vi "arduinoStop.vi"() -> (0 "error out":errorcluster)   [LabVIEW 2012]
uses:
  <vilib>/Instr/_visa.llb/Select Event Type.ctl
  GlobalArduino.vi
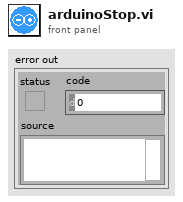
[diagram p1: front panel]
types:
  T1 = typedef "Select Event Type.ctl" = u32
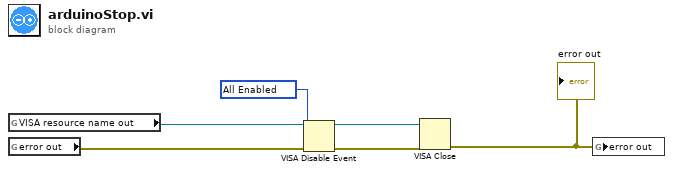
[diagram p0: block diagram]
diagram:
  w1 = T1 1073709055 items=["Service Request"=1073684491, "Trigger"=3221168138, "Clear"=1073684493, "VXI Signal"=1073684512, "VXI/VME Interrupt"=3221168161, "VXI/VME Sysfail"=1073684509, "VXI/VME Sysreset"=1073684510, "GPIB CIC"=1073684498, "GPIB Talk"=1073684499, "GPIB Listen"=1073684500, "PXI Interrupt"=1073684514, "Serial Break"=1073684515, "Serial TermChar"=1073684516, "Serial CTS"=1073684521, "Serial DSR"=1073684522, "Serial DCD"=1073684524, "Serial RI"=1073684526, "Serial Character"=1073684533, "USB Interrupt"=1073684535, "All Enabled"=1073709055] ("Event Type")
  n1 = global read "GlobalArduino.vi" "VISA resource name out"() -> (w3:refnum<visa-resource-name>)
  n2 = global read "GlobalArduino.vi" "error out"() -> (w4:errorcluster)
  n3 = VISA Disable Event(8:w4, 10:w1, 11:w3) -> (0:w5:errorcluster, 3:w2:refnum<visa-resource-name>)  [unwired: 1 out]
  n4 = VISA Close(VISA resource name=w2, error in (no error)=w5) -> (error out=w6:errorcluster)
  "error out" <- w6
  n5 = global write "GlobalArduino.vi" "error out"(w6) -> ()
